vi "Items (Type).vi"(8 "error in (no error)":errorcluster, 9 "EventToken":refnum<class "EventToken.lvclass">, 11 "EventBag in":refnum<class "EventBag.lvclass">) -> (0 "error out":errorcluster, 1 "Item found?":bool, 2 "Events":refnum<class "Event.lvclass">[](array[class]), 3 "EventBag out":refnum<class "EventBag.lvclass">)   [LabVIEW 2021, in "EventManagerLibrary.lvlib" / "EventBag.lvclass"]
uses:
  EventBag.lvclass
  EventToken/EventToken.lvclass
  EventObject/Event.lvclass
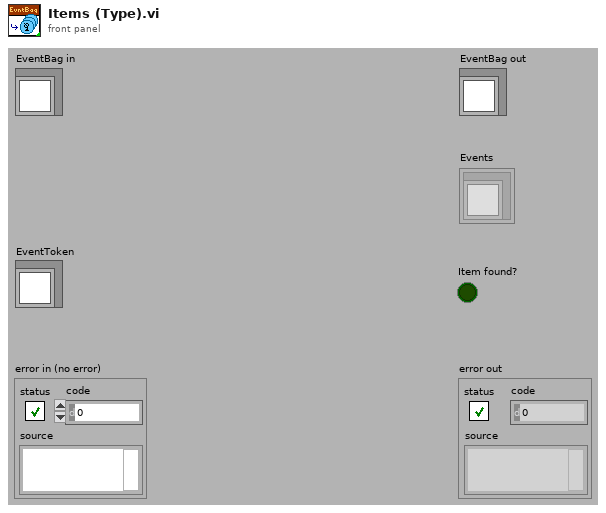
[diagram p1: front panel]
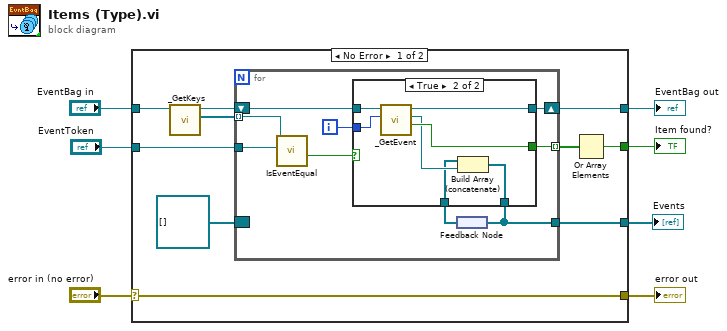
[diagram p0: block diagram]
diagram:
  n1 = case shown="No Error" "error in (no error)" {
    selector: "error in (no error)" -> [w9 w37]
    tunnel: [w9 w37] -> w6
    tunnel: [w14 w36] -> w4
    tunnel: "EventBag in" -> [w17 w36]
    tunnel: "EventToken" -> [w8 _]
    tunnel: [w10 _] -> w2
    tunnel: [w11 _] -> w1
    frame No Error {
      n2 = call "_GetKeys.vi"("EventBag in"=w17) -> ("Keys"=w16:refnum<class "EventToken.lvclass">[], "EventBag out"=w15:refnum<class "EventBag.lvclass">)  [unwired: 8 in, 1 out]
      n3 = for {
        tunnel: w16 -> [w19] mode=indexing
        shift-right: [w25] -> w14
        shift-left: w15 -> [w26]
        tunnel: [w24] -> w13 mode=indexing
        border: refnum<class "Event.lvclass">[] [] ("Events") -> [_]
        tunnel: [w22] -> w11
        tunnel: w8 -> [w18]
        i -> [w21]
        n4 = call-dynamic "IsEventEqual.vi"("EventToken"=w18, "EventToken in"=w19) -> ("Is Event Equal?"=w20:bool)  [unwired: 6 in, 3 out]
        n5 = feedback #1() -> (w23:refnum<class "Event.lvclass">[])
        n6 = case shown="True" w20 {
          tunnel: w26 -> [w28 w35]
          tunnel: [w28 w34] -> w25
          tunnel: [_ w33] -> w24
          tunnel: w23 -> [w27 w31]
          tunnel: [w27 w30] -> w22
          tunnel: w21 -> [_ w29]
          frame False {
          }
          frame True {
            n7 = call "_GetEvent.vi"("Index"=w29, "EventBag in"=w35) -> ("Item found?"=w33:bool, "Event"=w32:refnum<class "Event.lvclass">, "EventBag out"=w34:refnum<class "EventBag.lvclass">)  [unwired: 6 in, 1 out]
            n8 = Build Array (concatenate)(w31, w32) -> (w30:refnum<class "Event.lvclass">[])
          }
        }
        n9 = feedback-in #1(w22) -> ()
      }
      n10 = Or Array Elements(Boolean array=w13) -> (logical OR=w10:bool)
    }
    frame Error {
    }
  }
  "error out" <- w6
  "EventBag out" <- w4
  "Item found?" <- w2
  "Events" <- w1
